vi "CLUSTERSimpleS_AWrap.vi"() -> ()   [LabVIEW 2023]
doc: "This function takes a cluster that contains a DBL, string, and array of I32 (in that order) as input. It squares the value of the DBL, reverses the string, and doubles the value of each element in the array. The result is returned in output.\n\nFor information on the data types used for the DLL function, right-click on the Call Library Function node and choose Configure."
uses:
  CLF_Example.dll
panel:
  out "output":T1
  in  "input":T1={"DBL"=10.0, "String (50 Character Limit)"="abcd", "Array (50 Element Limit)"=[10, 100]}
  # "See the block diagram for more information."
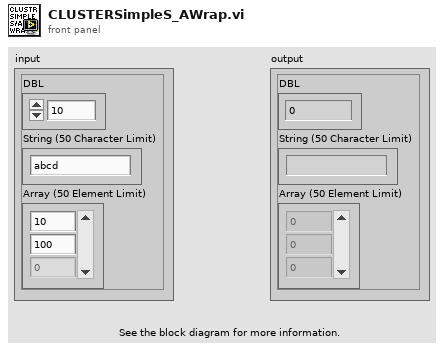
[diagram p1: front panel]
types:
  T1 = cluster{"DBL":dbl, "String (50 Character Limit)":string, "Array (50 Element Limit)":i32[]}
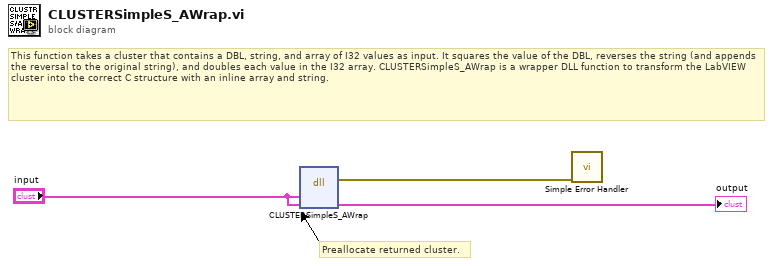
[diagram p0: block diagram]
diagram:
  # "Preallocate returned cluster."
  # "This function takes a cluster that contains a DBL, string, and array of I32 values as input. It squares the value of the DBL, reverses the string (and appends the reversal to the original string), and doubles each value in the I32 array. CLUSTERSimpleS_AWrap is a wrapper DLL function to transform the LabVIEW cluster into the correct C structure with an inline array and string."
  n1 = dll-call lib="c:/dev/_r/4/eng/lv-core/lvpostprocessingd/lv_mc_x86_64/dist_i386/examples/Connectivity/Libraries and Executables/DLL Calling VIs/CLF_Example**.*" fn="CLUSTERSimpleS_AWrap"("input"="input", "output"="input") -> (error out=w1:errorcluster, "output"=→"output":T1)  [unwired: 4 in, 2 out]
  n2 = call <vilib>:"Simple Error Handler.vi"("error in (no error)"=w1) -> ()  [unwired: 4 in, 5 out]
